vi "Track error states.vi"(0 "System":u16, 1 "Action(GET)":enum16{"GET", "Init", "New error state"}(ring), 7 "Loop":u16, 11 "error in (no error)":errorcluster, 12 "System type":variant, 13 "System Loops":variant[](array[variant])) -> (15 "error out":errorcluster)   [LabVIEW 2011]
uses:
  emi Lib/System 01/0 - General/S&E reporting/Private/_emi_ S&E Message.ctl
  emi Lib/System 01/0 - General/S&E reporting/Private/_emi_ S&E Message type.ctl
  <vilib>/Utility/VariantDataType/GetNumericInfo.vi
  <vilib>/Utility/VariantDataType/VariantType.lvlib
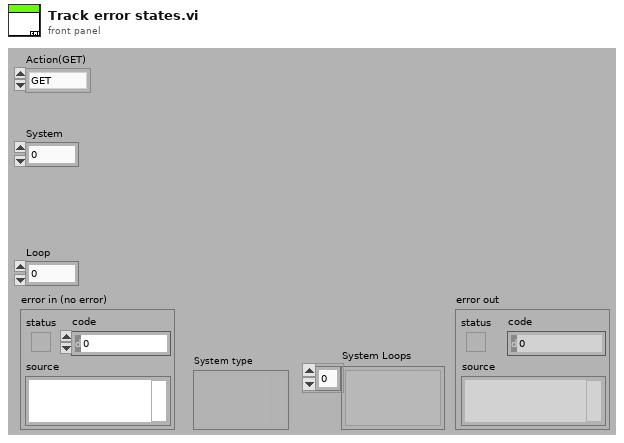
[diagram p1: front panel]
types:
  T1 = typedef "_emi_ S&E Message.ctl" = cluster{"Type":T2, "Originate time":dbl, "System":u8, "Loop":u16, "Sub ID":u16, "Elevated priority":bool, "E&S Message content":variant}
  T2 = typedef "_emi_ S&E Message type.ctl" = enum16{"Error/Warning", "Note", "Debug", "Event", "Alarm Analog", "Alarm Digital", "Annotation"}
  T3 = typedef "VariantType.lvlib/Type.ctl" = enum8{"Invalid Type", "Void", "I8", "I16", "I32", "I64", "U8", "U16", "U32", "U64", "Single Float", "Double Float", "Extended Float", "Single Complex", "Double Complex", "Extended Complex", "Enum U8", "Enum U16", "Enum U32", "Enum U64", "Single Float With Unit", "Double Float With Unit", "Extended Float With Unit", "Single Complex with Unit", "Double Complex with Unit", "Extended Complex with Unit", "Boolean", "String", "Path", "Picture", "Tag", "Array", "Cluster", "Variant", "LV Variant", "Waveform", "Timestamp", "Digital Waveform", "Digital Data", "ExpressData", "Refnum", "External Data", "VI", "Poly VI", "LabVIEW Class Instance", "Fixed Point"}
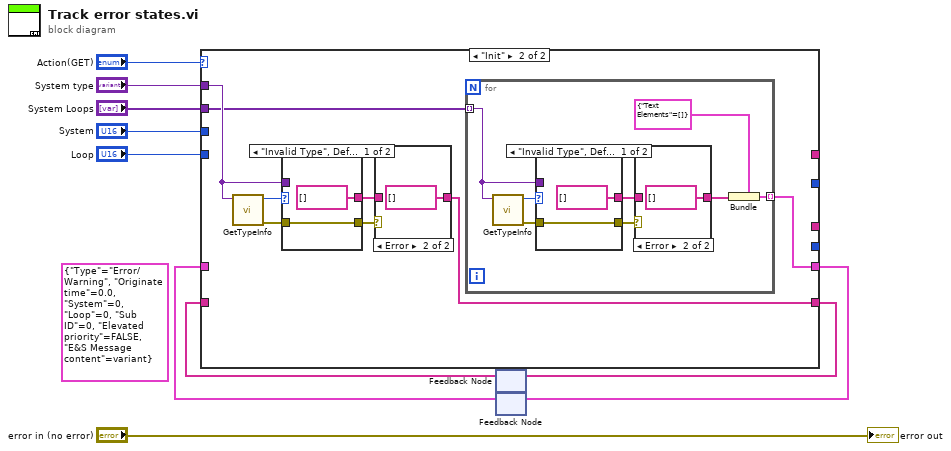
[diagram p0: block diagram]
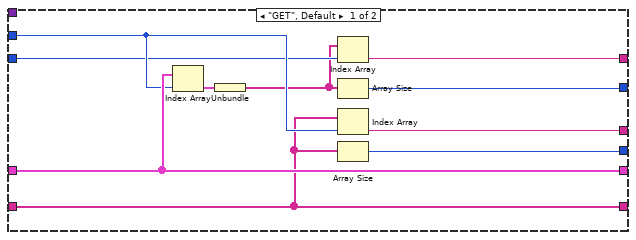
[diagram p2: hidden frame]
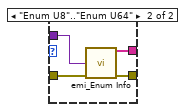
[diagram p4: hidden frame]
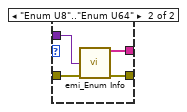
[diagram p6: hidden frame]
diagram:
  (unwired) T1 {"Type"=enum."Error/Warning", "Originate time"=0.0, "System"=0, "Loop"=0, "Sub ID"=0, "Elevated priority"=FALSE, "E&S Message content"=variant} ("E&S Message")
  n1 = feedback #1() -> (w1:string[])  [unwired: 1 in]
  n2 = feedback #2() -> (w2:cluster{"Text Elements":string[]}[])  [unwired: 1 in]
  n3 = case shown="\"Init\"" "Action(GET)" {
    tunnel: [w19 w21] -> w8
    tunnel: w2 -> [w19 _]
    tunnel: "System type" -> [_ w26]
    tunnel: "System Loops" -> [_ w22]
    tunnel: "System" -> [w18 _]
    tunnel: "Loop" -> [w16 _]
    tunnel: [w12 w23] -> w3
    tunnel: w1 -> [w12 _]
    tunnel: [w20 _] -> _
    tunnel: [w15 _] -> _
    tunnel: [w13 _] -> _
    tunnel: [w11 _] -> _
    frame "GET", Default {
      n4 = Index Array(array=w19, index=w18) -> (element=w17:cluster{"Text Elements":string[]})
      n5 = Unbundle(w17) -> ("Text Elements"=w14:string[])
      n6 = Index Array(array=w14, index=w16) -> (element=w15:string)
      n7 = Array Size(array=w14) -> (size(s)=w13:i32)
      n8 = Index Array(array=w12, index=w18) -> (element=w20:string)
      n9 = Array Size(array=w12) -> (size(s)=w11:i32)
    }
    frame "Init" {
      n10 = call <vilib>:"GetTypeInfo.vi"("Variant"=w26) -> ("error out"=w27:errorcluster, "Type Enum"=w28:T3)  [unwired: 6 in, 3 out]
      n11 = case shown="\"Invalid Type\", Default" w28 {
        tunnel: w26 -> [_ w52]
        tunnel: w27 -> [w47 w51]
        tunnel: [string[] [] ("Text Elements") w50] -> w24
        tunnel: [w47 w49] -> w25
        frame "Invalid Type", Default {
        }
        frame "Enum U8".."Enum U64" {
          n12 = call "emi_Enum Info.vi"("Enum"=w52, "error in (no error)"=w51) -> ("Text Elements"=w50:string[], "error out"=w49:errorcluster)  [unwired: 10 in, 2 out]
        }
      }
      n13 = case shown="Error" w25 {
        tunnel: [w45 string[] [] ("Text Elements")] -> w23
        tunnel: w24 -> [w45 _]
        frame No Error {
        }
        frame Error {
        }
      }
      n14 = for {
        tunnel: w22 -> [w32] mode=indexing
        tunnel: [w29] -> w21 mode=indexing
        n15 = call <vilib>:"GetTypeInfo.vi"("Variant"=w32) -> ("error out"=w34:errorcluster, "Type Enum"=w33:T3)  [unwired: 6 in, 3 out]
        n16 = case shown="\"Invalid Type\", Default" w33 {
          tunnel: w32 -> [_ w44]
          tunnel: w34 -> [w39 w43]
          tunnel: [string[] [] ("Text Elements") w42] -> w36
          tunnel: [w39 w41] -> w35
          frame "Invalid Type", Default {
          }
          frame "Enum U8".."Enum U64" {
            n17 = call "emi_Enum Info.vi"("Enum"=w44, "error in (no error)"=w43) -> ("Text Elements"=w42:string[], "error out"=w41:errorcluster)  [unwired: 10 in, 2 out]
          }
        }
        n18 = case shown="Error" w35 {
          tunnel: [w37 string[] [] ("Text Elements")] -> w31
          tunnel: w36 -> [w37 _]
          frame No Error {
          }
          frame Error {
          }
        }
        n19 = Bundle(cluster=cluster{"Text Elements":string[]} {"Text Elements"=[]} ("output cluster"), "Text Elements"=w31) -> (w29:cluster{"Text Elements":string[]})
      }
    }
  }
  n20 = feedback-in #1(w3) -> ()
  n21 = feedback-in #2(w8) -> ()
  "error out" <- "error in (no error)"
